vi "offset_WFm.vi"(2 "Controls Cluster":T4 {"C1 vertical coupling / V" items=["AC", "DC", "Ground"]; "C2 vertical coupling / V" items=["AC", "DC", "Ground"]; "Trigger slope" items=["Positive", "Negative"]}, 7 "WFm":waveform(dbl)={"t0"=timestamp(0 s since 1904-01-01), "dt"=0.0, "Y"=[]} caption="wfm") -> (4 "WFm Offset / s":dbl, 8 "Offset WFm":waveform(dbl))   [LabVIEW 2023]
uses:
  <instrlib>/niScope/Controls/niScope trigger slope.ctl
  <instrlib>/niScope/Controls/niScope trigger source.ctl
  <instrlib>/niScope/Controls/niScope vertical coupling.ctl
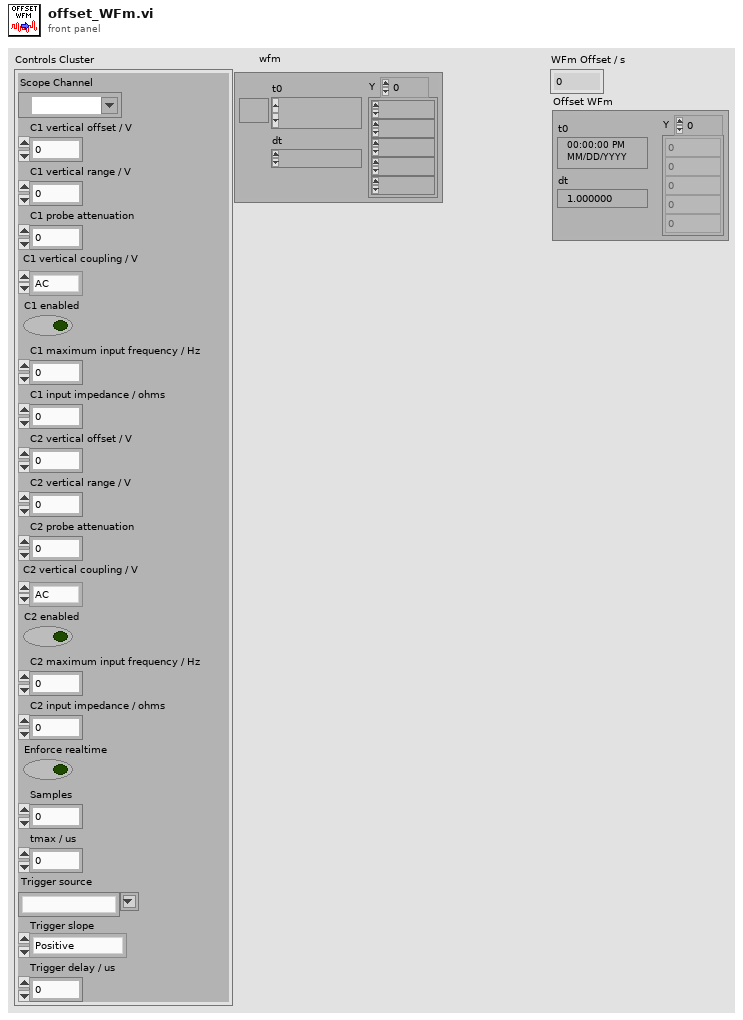
[diagram p1: front panel]
types:
  T1 = typedef "niScope vertical coupling.ctl" = i32
  T2 = typedef "niScope trigger source.ctl" = string
  T3 = typedef "niScope trigger slope.ctl" = i32
  T4 = cluster{"Scope Channel":refnum<k15>, "C1 vertical offset / V":dbl, "C1 vertical range / V":dbl, "C1 probe attenuation":dbl, "C1 vertical coupling / V":T1, "C1 enabled":bool, "C1 maximum input frequency / Hz":dbl, "C1 input impedance / ohms":u32, "C2 vertical offset / V":dbl, "C2 vertical range / V":dbl, "C2 probe attenuation":dbl, "C2 vertical coupling / V":T1, "C2 enabled":bool, "C2 maximum input frequency / Hz":dbl, "C2 input impedance / ohms":u32, "Enforce realtime":bool, "Samples":i64, "tmax / us ":dbl, "Trigger source":T2, "Trigger slope":T3, "Trigger delay / us":dbl}
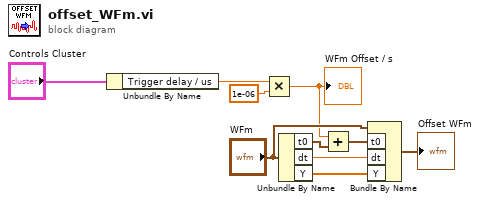
[diagram p0: block diagram]
diagram:
  n1 = Unbundle By Name("Controls Cluster") -> ("Trigger delay / us"=w9:dbl)
  n2 = Multiply(x=w9, y=1e-06) -> (x*y=w2:dbl)
  "WFm Offset / s" <- w2
  n3 = Unbundle By Name("WFm") -> ("t0"=w7:timestamp, "dt"=w4:dbl, "Y"=w5:dbl[])
  n4 = Add(x=w2, y=w7) -> (x+y=w6:timestamp)
  n5 = Bundle By Name(cluster="WFm", "t0"=w6, "dt"=w4, "Y"=w5) -> (→"Offset WFm":waveform(dbl))
